vi "CtrlTreeAddItem.vi"   [LabVIEW 2021]
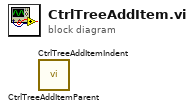
[diagram p0: block diagram]
diagram:
  n1 = call "CtrlTreeAddItemParent.vi"() -> ()  [unwired: 13 in, 3 out]
  n2 = call "CtrlTreeAddItemIndent.vi"() -> ()  [unwired: 13 in, 3 out]
